vi "InteractWithScrollBar (SubVI).vi"(10 "element":i32, 11 "Table in":refnum<vi>) -> ()   [LabVIEW 2017]
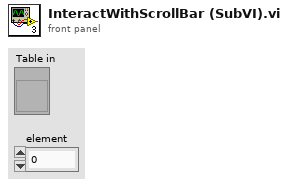
[diagram p1: front panel]
types:
  T1 = typedef "LVRowAndColumnUnsignedTypeDef.ctl" = cluster{"Row":u32, "Column":u32}
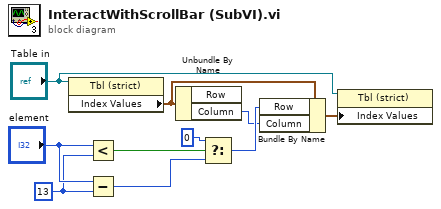
[diagram p0: block diagram]
diagram:
  w8 = 13 ("y")
  n1 = property on="Property Node" class="Tbl (strict)"(reference="Table in") -> ("Index Values"=w3:T1)  [unwired: 1 in, 2 out]
  n2 = Less?(x="element", y=w8) -> (x < y?=w5:bool)
  n3 = Subtract(x="element", y=w8) -> (x-y=w10:i32)
  n4 = Unbundle By Name(w3) -> ("Column"=w2:u32)  [unwired: 1 out]
  n5 = Select(t=0 ("y"), s=w5, f=w10) -> (s? t:f=w7:i32)
  n6 = Bundle By Name(cluster=w3, "Row"=w7, "Column"=w2) -> (w4:T1)
  n7 = property on="Property Node" class="Tbl (strict)"(reference="Table in", "Index Values"=w4) -> ()  [unwired: 1 in, 2 out]
